vi "Center Calculated Distance.vi"(11 "Normalized Rect":T1) -> (2 "Distance (ft)":dbl)   [LabVIEW 2015]
panel:
  out "Distance Right (ft)":dbl
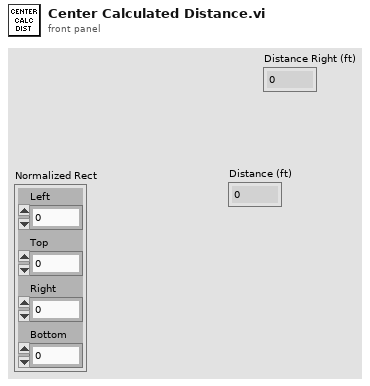
[diagram p1: front panel]
types:
  T1 = cluster{"Left":dbl, "Top":dbl, "Right":dbl, "Bottom":dbl}
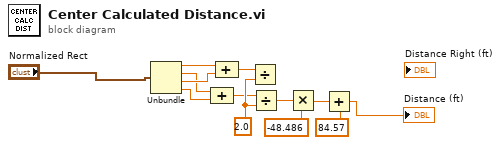
[diagram p0: block diagram]
diagram:
  w9 = 2.0
  n1 = Unbundle("Normalized Rect") -> ("Left"=w13:dbl, "Top"=w10:dbl, "Right"=w12:dbl, "Bottom"=w11:dbl)
  n2 = Compound Arithmetic op=ADD(w10, w11) -> (w7:dbl)
  n3 = Compound Arithmetic op=ADD(w13, w12) -> (w8:dbl)
  n4 = Divide(x=w8, y=w9) -> ()  [unwired: 1 out]
  n5 = Divide(x=w7, y=w9) -> (x/y=w5:dbl)
  n6 = Multiply(x=w5, y=-48.486) -> (x*y=w3:dbl)
  n7 = Add(x=w3, y=84.57) -> (x+y=→"Distance (ft)":dbl)
